vi "Off_Asc&DTCE_K2.vi"(2 "Timeout (ms)":i32=40000000, 3 "connection ID in":refnum<k5>) -> (0 "Timeout (ms) 2":i32=40000000, 1 "connection ID out":refnum<k5>)   [LabVIEW 2016]
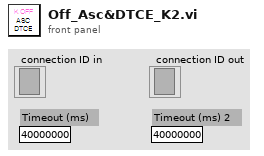
[diagram p1: front panel]
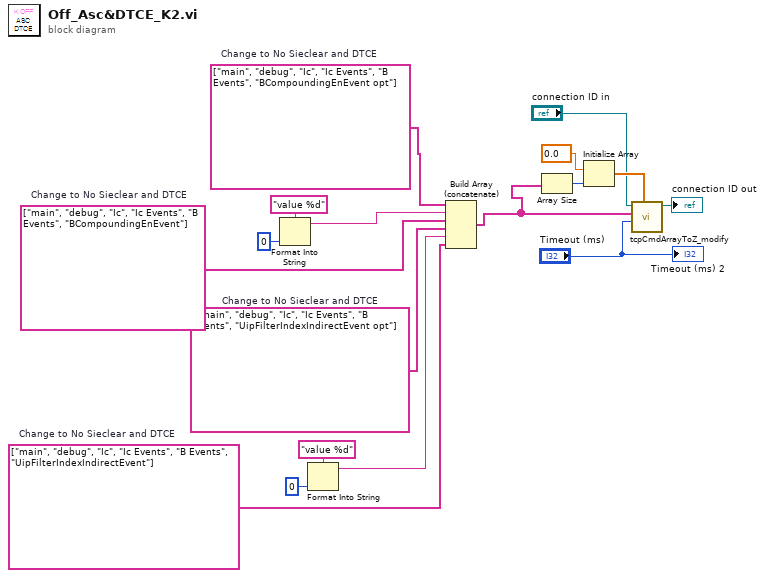
[diagram p0: block diagram]
diagram:
  w2 = string[] ["main", "debug", "Ic", "Ic Events", "B Events", "UipFilterIndexIndirectEvent"]  # Change to No Sieclear and DTCE
  w3 = string[] ["main", "debug", "Ic", "Ic Events", "B Events", "BCompoundingEnEvent"]  # Change to No Sieclear and DTCE
  w7 = string[] ["main", "debug", "Ic", "Ic Events", "B Events", "UipFilterIndexIndirectEvent opt"]  # Change to No Sieclear and DTCE
  w11 = string[] ["main", "debug", "Ic", "Ic Events", "B Events", "BCompoundingEnEvent opt"]  # Change to No Sieclear and DTCE
  n1 = Format Into String(format string="value %d", 0 ("입력 1")) -> (resulting string=w9:string)  [unwired: 2 in, 1 out]
  n2 = Format Into String(format string="value %d", 0 ("입력 1")) -> (resulting string=w4:string)  [unwired: 2 in, 1 out]
  n3 = Build Array (concatenate)(w11, w9, w3, w7, w4, w2) -> (w1:string[])
  n4 = Array Size(array=w1) -> (size(s)=w17:i32)
  n5 = Initialize Array(0.0 ("element"), w17) -> (w15:dbl[])
  n6 = call "tcpCmdArrayToZ_modify.vi"("Delay (sec)"=w15, "Timeout (ms)"="Timeout (ms)", "Command array"=w1, "connection ID in"="connection ID in") -> ("connection ID out"=→"connection ID out":refnum<k5>)  [unwired: 3 in, 4 out]
  "Timeout (ms) 2" <- "Timeout (ms)"
